vi "diming light.vi"() -> ()   [LabVIEW 2020]
doc: "Manually blink and LED attached to a digital output channel of a LINX device by clicking and LED control in LabVIEW."
uses:
  <vilib>/MakerHub/LINX/Public/Peripherals/PWM/PWM Set Duty Cycle 1 Chan.vi
  <vilib>/MakerHub/LINX/Public/Utilities/Open Serial.vi
  <vilib>/MakerHub/LINX/Public/Peripherals/PWM/PWM Set Duty Cycle N Chans.vi
  <vilib>/MakerHub/LINX/LMH-LINX.lvlib
panel:
  in  "AI Channel for photocell":u8
  out "Loop Rate (Hz)":u32=69
  out "PWM Out (0-1)":dbl(knob) scale=0.0..1.0 scale format="%.2f"
  in  "LED Channel (digital)":u8=9
  in  "Serial Port":refnum<visa-resource-name>="COM9"
  in  "Stop Button":bool
  # "This example was created by combining code from LINX - Blink (Simple), LINX - PWM 1 Channel, and LINX - Photocell VIs\nIn addition, the circuitry for how to control a DC motor was modified from the example in:\nElegoo The Most Complete Starter Kit for UNO V2.0.2020.4.3\\English\\Part 2 Module Learning\\2.23 DC Motors"
  # "LINX Device Settings"
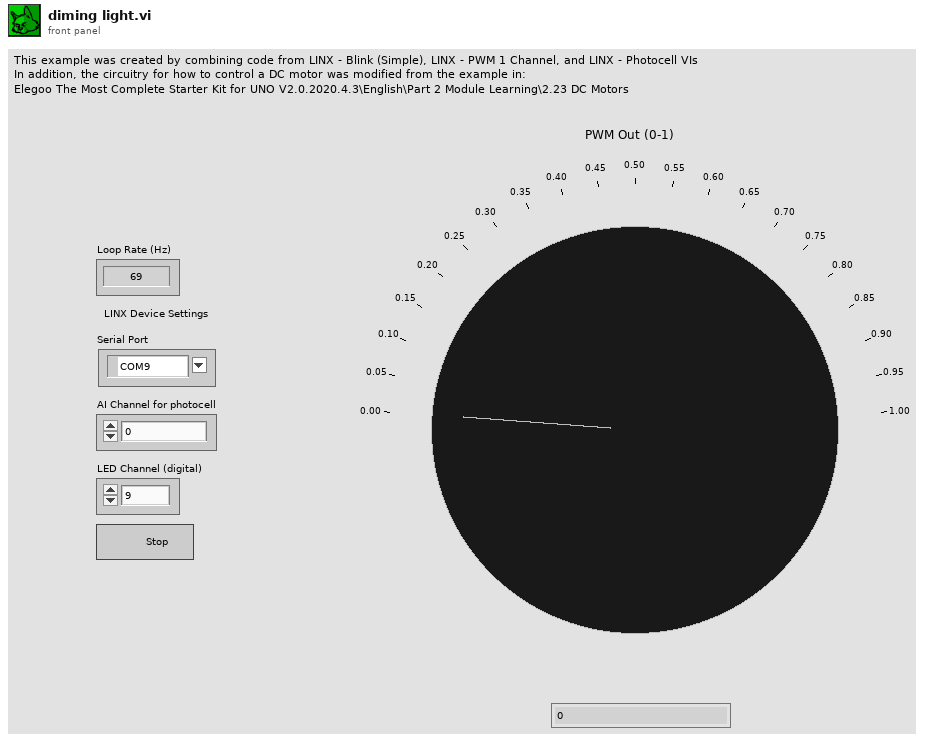
[diagram p1: front panel]
types:
  T1 = typedef "LMH-LINX.lvlib/LINX Ref.ctl" = cluster{"IO":T2, "Interface":T3, "LINX Device Config":T4}
  T2 = typedef "LMH-LINX.lvlib/Platform.ctl" = enum16{"Remote", "Local"}
  T3 = typedef "LMH-LINX.lvlib/Interface.ctl" = enum16{"Serial", "TCP"}
  T4 = typedef "LMH-LINX.lvlib/Device.lvlib/LINX Device Config.ctl" = cluster{"Interface":T3, "COM Port":refnum<visa-resource-name>, "TCP Configuration":T5, "Device Family":u8, "Device ID":u8, "Device Name":string, "TCP Ref":refnum<k5>, "Channels":T6}
  T5 = typedef "LMH-LINX.lvlib/Device.lvlib/TCP Config.ctl" = cluster{"IP Address":string, "Port":u16}
  T6 = typedef "LMH-LINX.lvlib/Channels.ctl" = cluster{"DI":u8[], "DO":u8[], "AI":u8[], "AO":u8[], "PWM":u8[], "QE":u8[], "UART":u8[], "I2C 2":u8[], "SPI":u8[], "CAN":u8[], "Servo":u8[], "AI Ref (V)":dbl, "AI Resolution (Bits)":u8, "AO Ref (V)":dbl, "AO Resolution (Bits)":u8}
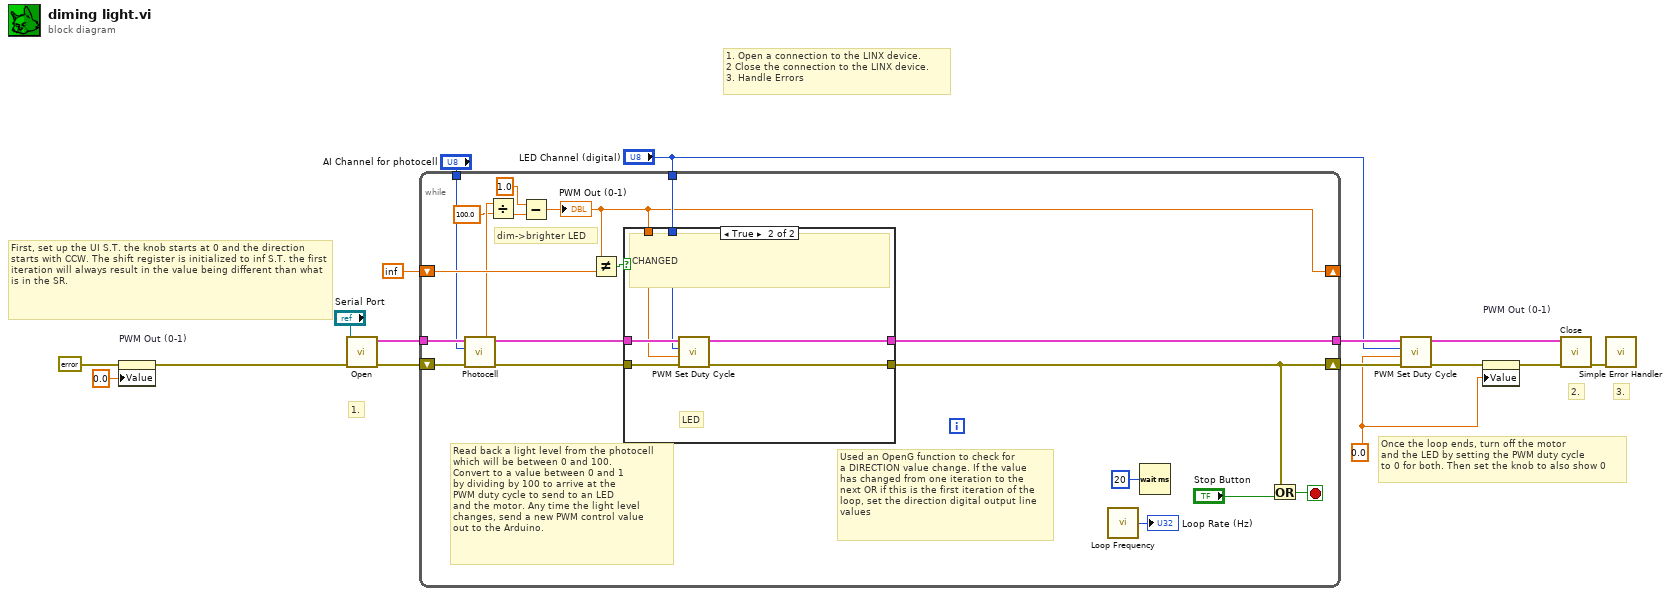
[diagram p0: block diagram]
diagram:
  w6 = 0.0
  # "Once the loop ends, turn off the motor\nand the LED by setting the PWM duty cycle\nto 0 for both. Then set the knob to also show 0"
  # "First, set up the UI S.T. the knob starts at 0 and the direction starts with CCW. The shift register is initialized to inf S.T. the first iteration will always result in the value being different than what is in the SR."
  # "1. Open a connection to the LINX device.\n2 Close the connection to the LINX device.\n3. Handle Errors"
  # "3."
  # "2."
  # "1."
  n1 = property on="PWM Out (0-1)" class="Knob (strict)"(error in=errorcluster {"status"=FALSE, "code"=0, "source"=""} ("Error In"), "Value"=0.0) -> (error out=w1:errorcluster)  [unwired: 1 in, 1 out]
  n2 = call-poly <vilib>:"Open.vi"("Error In"=w1, "Serial Port"="Serial Port") -> ("Error Out"=w15:errorcluster, "LINX Resource"=w16:T1)  [unwired: 7 in, 1 out]
  n3 = while {
    tunnel: w16 -> [w26]
    tunnel: [w20] -> w8
    shift-right: [w21] -> w9
    shift-left: w15 -> [w28]
    tunnel: "LED Channel (digital)" -> [w32]
    shift-right: [w17] -> _
    shift-left: inf -> [w31]
    tunnel: "AI Channel for photocell" -> [w25]
    stop <- w35 stop-if-true
    # "dim->brighter LED"
    # "Used an OpenG function to check for\na DIRECTION value change. If the value\nhas changed from one iteration to the\nnext OR if this is the first iteration of the\nloop, set the direction digital output line\nvalues"
    # "Read back a light level from the photocell\nwhich will be between 0 and 100.\nConvert to a value between 0 and 1\nby dividing by 100 to arrive at the\nPWM duty cycle to send to an LED\nand the motor. Any time the light level\nchanges, send a new PWM control value\nout to the Arduino."
    n4 = call <vilib>:"Photocell.vi"("Error In"=w28, "AI Channel"=w25, "LINX Resource"=w26) -> ("Error Out"=w27:errorcluster, "Value (0-100)"=w23:dbl, "LINX Resource"=w24:T1)  [unwired: 6 in]
    n5 = Divide(x=w23, y=100.0) -> (x/y=w18:dbl)
    n6 = Subtract(x=1.0, y=w18) -> (x-y=w17:dbl)
    "PWM Out (0-1)" <- w17
    n7 = Not Equal?(x=w17, y=w31) -> (x != y?=w30:bool)
    n8 = case shown="True" w30 {
      tunnel: w24 -> [w37 w43]
      tunnel: [w37 w39] -> w20
      tunnel: w27 -> [w36 w42]
      tunnel: [w36 w38] -> w21
      tunnel: w17 -> [_ w40]
      tunnel: w32 -> [_ w41]
      frame False {
        # "SAME"
      }
      frame True {
        # "LED"
        # "CHANGED"
        n9 = call-poly <vilib>:"PWM Set Duty Cycle.vi"("Error In"=w42, "Duty Cycle (0-1)"=w40, "PWM Channel"=w41, "LINX Resource"=w43) -> ("Error Out"=w38:errorcluster, "LINX Resource"=w39:T1)  [unwired: 6 in]
      }
    }
    n10 = call <vilib>:"Loop Frequency.vi"() -> ("Loop Rate (Hz)"=→"Loop Rate (Hz)":u32)
    n11 = Wait (ms)(milliseconds to wait=u32 20) -> ()  [unwired: 1 out]
    n12 = Or(x=w21, y="Stop Button") -> (x .or. y?=w35:bool)
  }
  n13 = call-poly <vilib>:"PWM Set Duty Cycle.vi"("Error In"=w9, "Duty Cycle (0-1)"=w6, "PWM Channel"="LED Channel (digital)", "LINX Resource"=w8) -> ("Error Out"=w2:errorcluster, "LINX Resource"=w4:T1)  [unwired: 6 in]
  n14 = property on="PWM Out (0-1)" class="Knob (strict)"(error in=w2, "Value"=w6) -> (error out=w3:errorcluster)  [unwired: 1 in, 1 out]
  n15 = call <vilib>:"Close.vi"("Error In"=w3, "LINX Resource"=w4) -> ("Error Out"=w13:errorcluster)  [unwired: 9 in]
  n16 = call <vilib>:"Simple Error Handler.vi"("error in (no error)"=w13) -> ()  [unwired: 4 in, 5 out]
